vi "Pre Launch Init.vi"(11 "Multiharp in":refnum<class "Multiharp.lvclass">) -> (0 "error out":errorcluster, 3 "Multiharp out":refnum<class "Multiharp.lvclass">)   [LabVIEW 2023, in "Multiharp.lvlib" / "Multiharp.lvclass"]
doc: "(<B>Filename</B>: Actor Framework.lvlib:Actor.lvclass:Pre Launch Init.vi)\n\nDefines behavior that occurs after the Launch Nested Actor method is invoked but before the actor's Actor Core method begins running.\n\nBy default, this method does nothing. A descendant class may override it to define behavior."
uses:
  Multiharp.lvclass
  <vilib>/ActorFramework/Actor/Actor.lvclass
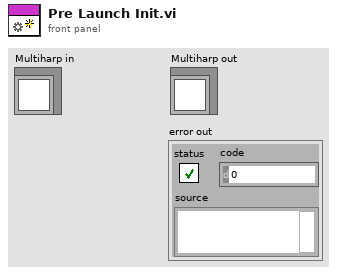
[diagram p1: front panel]
types:
  T1 = cluster{"Acquiring":bool, "tacq":i32, "Scanning":bool, "Max Triggers":i32, "Coincidence Window":dbl, "file path":path, "Coincidence Delays":dbl[]}
  T2 = cluster{"HistoOn/Off":bool, "ActualHistoLe":i32, "tacq":i32}
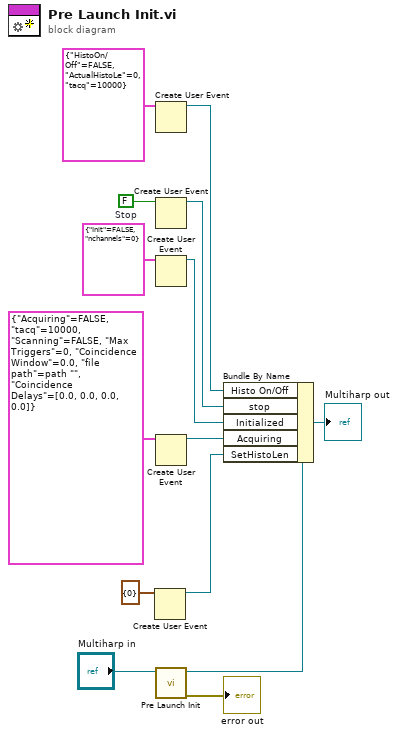
[diagram p0: block diagram]
diagram:
  w9 = FALSE  # Stop
  n1 = Create User Event(user event datatype=cluster{"ActualHistoLe":i32} {"ActualHistoLe"=0} ("event data")) -> (user event=w2:refnum<user-event>)  [unwired: 1 in, 1 out]
  n2 = Create User Event(user event datatype=T2 {"HistoOn/Off"=FALSE, "ActualHistoLe"=0, "tacq"=10000} ("Histo On/Off")) -> (user event=w7:refnum<user-event>)  [unwired: 1 in, 1 out]
  n3 = Create User Event(user event datatype=w9) -> (user event=w10:refnum<user-event>)  [unwired: 1 in, 1 out]
  n4 = Create User Event(user event datatype=cluster{"Init":bool, "nchannels":i32} {"Init"=FALSE, "nchannels"=0} ("Histo On/Off")) -> (user event=w6:refnum<user-event>)  [unwired: 1 in, 1 out]
  n5 = Create User Event(user event datatype=T1 {"Acquiring"=FALSE, "tacq"=10000, "Scanning"=FALSE, "Max Triggers"=0, "Coincidence Window"=0.0, "file path"=path "", "Coincidence Delays"=[0.0, 0.0, 0.0, 0.0]} ("Histo On/Off")) -> (user event=w4:refnum<user-event>)  [unwired: 1 in, 1 out]
  n6 = call-parent "Pre Launch Init.vi"("Actor in"="Multiharp in") -> ("error out"=→"error out":errorcluster, "Actor out"=w12:refnum<class "Multiharp.lvclass">)  [unwired: 9 in]
  n7 = Bundle By Name(cluster=w12, "Histo On/Off"=w7, "stop"=w10, "Initialized"=w6, "Acquiring"=w4, "SetHistoLen"=w2) -> (→"Multiharp out":refnum<class "Multiharp.lvclass">)
